vi "Close.vi"(8 "Error In":errorcluster, 11 "EZ430-Chronos Config":T1) -> (0 "Error Out":errorcluster)   [LabVIEW 2011, in "LVH-EZ430.lvlib"]
doc: "Close the connection to the EZ430-Chronos."
uses:
  LVH-EZ430.lvlib
  Private/Type Defs/EZ430-Chronos Config.ctl
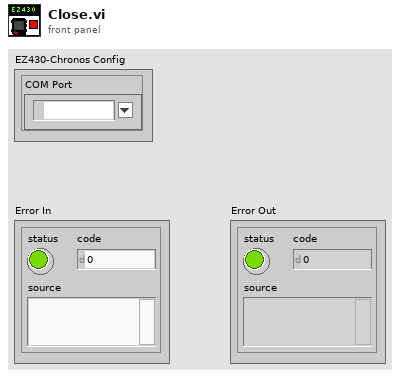
[diagram p1: front panel]
types:
  T1 = typedef "LVH-EZ430.lvlib/EZ430-Chronos Config.ctl" = cluster{"COM Port":refnum<visa-resource-name>}
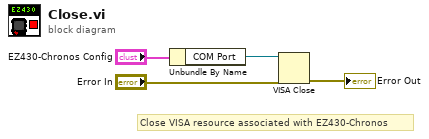
[diagram p0: block diagram]
diagram:
  # "Close VISA resource associated with EZ430-Chronos"
  n1 = Unbundle By Name("EZ430-Chronos Config") -> ("COM Port"=w1:refnum<visa-resource-name>)
  n2 = VISA Close(VISA resource name=w1, error in (no error)="Error In") -> (error out=→"Error Out":errorcluster)
